vi "SMTP_email_MultiAttach_Authenticated.vi"(0 "Recipients":string[](array[string]), 1 "SMTPServer:Port":string, 2 "From Address":string, 5 "Subject":string, 7 "Message":string, 9 "Attachments":path[](array[path]), 11 "Error In":errorcluster) -> (15 "Error Out":errorcluster)   [LabVIEW 2016]
uses:
  <vilib>/smtpClient/Set Message Text.vi
  <vilib>/smtpClient/LabVIEWSMTPClient.lvlib
panel:
  in  "Use Secure Connection (TLS\\SSL)":bool
  in  "Password":string
  in  "Username":string
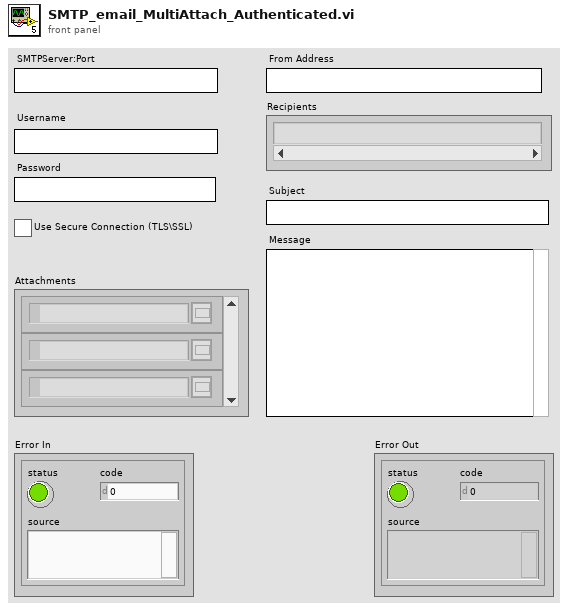
[diagram p1: front panel]
types:
  T1 = typedef "LabVIEWSMTPClient.lvlib/SmtpClientHandle.ctl" = refnum<k1>
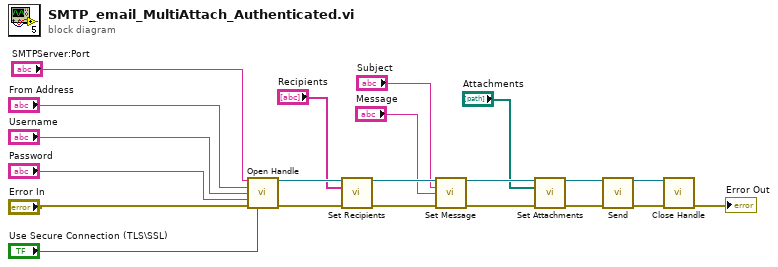
[diagram p0: block diagram]
diagram:
  n1 = call <vilib>:"Open Handle.vi"("server address"="SMTPServer:Port", "from"="From Address", "username"="Username", "password"="Password", "error in (no error)"="Error In", "use TLS (false)"="Use Secure Connection (TLS\\SSL)") -> ("handle out"=w17:T1, "error out"=w16:errorcluster)  [unwired: 8 in]
  n2 = call <vilib>:"Set Recipients.vi"("handle in"=w17, "to"="Recipients", "error in (no error)"=w16) -> ("handle out"=w15:T1, "error out"=w14:errorcluster)  [unwired: 11 in]
  n3 = call-poly <vilib>:"Set Message.vi"("handle in"=w15, "subject"="Subject", "plain text message"="Message", "error in (no error)"=w14) -> ("handle out"=w9:T1, "error out"=w8:errorcluster)  [unwired: 10 in]
  n4 = call <vilib>:"Set Attachments.vi"("handle in"=w9, "attachments"="Attachments", "error in (no error)"=w8) -> ("handle out"=w7:T1, "error out"=w6:errorcluster)  [unwired: 11 in]
  n5 = call <vilib>:"Send.vi"("handle in"=w7, "error in (no error)"=w6) -> ("handle out"=w12:T1, "error out"=w13:errorcluster)  [unwired: 11 in, 1 out]
  n6 = call <vilib>:"Close Handle.vi"("handle in"=w12, "error in (no error)"=w13) -> ("error out"=→"Error Out":errorcluster)  [unwired: 12 in, 1 out]
